vi "CallMatLabFunction.vi"(8 "error in (no error)":errorcluster) -> (0 "error out":errorcluster, 3 "Chirp Parametesr":T1)   [LabVIEW 2017]
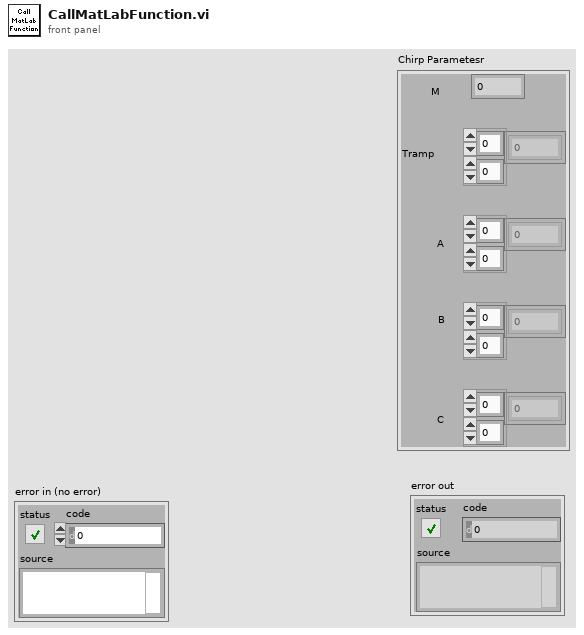
[diagram p1: front panel]
types:
  T1 = cluster{"M ":dbl, "Tramp":dbl[][], "A":dbl[][], "B":dbl[][], "C":dbl[][]}
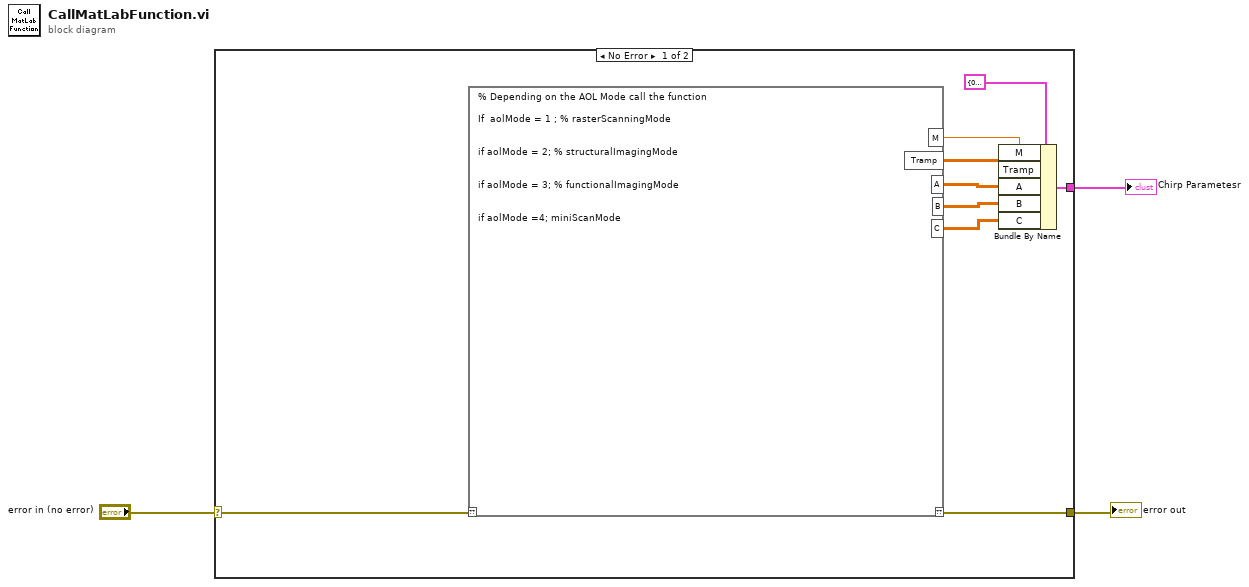
[diagram p0: block diagram]
diagram:
  n1 = case shown="No Error" "error in (no error)" {
    selector: "error in (no error)" -> [w11 w13]
    tunnel: [w12 w13] -> w2
    tunnel: [w4 _] -> w1
    frame No Error {
      n2 = script code="% Depending on the AOL Mode call the function\n\nIf  aolMode = 1 ; % rasterScanningMode\n\n    \nif aolMode = 2; % structuralImagingMode\n\n\nif aolMode = 3; % functionalImagingMode\n\n\nif aolMode =4; miniScanMode"("??"=w11) -> ("??"=w12:errorcluster, "M"=w5:dbl, "Tramp"=w6:dbl[][], "A"=w7:dbl[][], "B"=w8:dbl[][], "C"=w9:dbl[][])
      n3 = Bundle By Name(cluster=T1 {"M "=0.0, "Tramp"=[], "A"=[], "B"=[], "C"=[]} ("Chirp Parametesr"), "M"=w5, "Tramp"=w6, "A"=w7, "B"=w8, "C"=w9) -> (w4:T1)
    }
    frame Error {
    }
  }
  "Chirp Parametesr" <- w1
  "error out" <- w2
